vi "CAN GPS Werte.vi"() -> (2 "CAN data":T1[](array[typedef])=[{"timestamp"=timestamp(0 s since 1904-01-01), "payload"=[0, 2, 3, 4, 5, 6, 7, 8], "identifier"=2, "type"=0, "extended?"=FALSE, "echo?"=FALSE}, {"timestamp"=timestamp(0 s since 1904-01-01), "payload"=[0, 1, 2, 3, 4, 5, 6, 7], "identifier"=3, "type"=0, "extended?"=FALSE, "echo?"=FALSE}] {"payload" format="%x"; "timestamp" format="%<%.7X\n%x>T"; "type" items=["CAN Data"=0, "CAN Remote"=1, "CAN Bus Error"=2, "CAN 2.0 Data"=8, "CAN FD Data"=16, "CAN FD+BRS Data"=24, "J1939 Data"=192, "Delay"=224, "Log Trigger"=225, "Start Trigger"=226]; "identifier" format="%x"})   [LabVIEW 2020]
uses:
  <vilib>/xnet/xnet.llb/XNET Frame CAN.ctl
  <vilib>/xnet/xnet.llb/XNET Frame Type CAN.ctl
  FGV CAN Daten Aktionen.ctl
  Allgemein/Aktion FGV GPS.ctl
  CAN Interface.lvlib
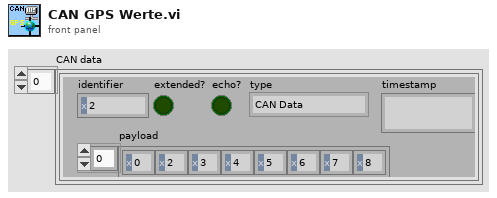
[diagram p1: front panel]
types:
  T1 = typedef "XNET Frame CAN.ctl" = cluster{"timestamp":timestamp, "payload":u8[], "identifier":u32, "type":T2, "extended?":bool, "echo?":bool}
  T2 = typedef "XNET Frame Type CAN.ctl" = u8
  T3 = typedef "Allgemein.lvlib/Aktion FGV GPS.ctl" = enum16{"lesen", "schreiben"}
  T4 = typedef "CAN Interface.lvlib/FGV CAN Daten Aktionen.ctl" = enum16{"lesen", "Daten", "Konfig", "laden", "speichern", "Status"}
  T5 = typedef "Allgemein.lvlib/GPS Daten cRio.ctl" = cluster{"GPS Zeit":string, "Breitengrad":string, "Längengrad":string, "Qualität":string, "Anzahl Satelliten":string, "Genauigkeit":string, "Höhe":string, "Höhe Geoid-Ellipsoid":string, "Geschwindigkeit":string, "Kurs wahr":string, "Kurs magnetisch":string, "Bewegungsrichtung":string, "Datum":string, "Breitengrad Roh":string, "Längengrad Roh":string}
  T6 = typedef "CAN Konfig.lvlib/Konfig Daten PC.ctl" = cluster{"Baude Rate":T7, "COM state":u8, "Frame-ID FTIR Start":u32, "Frame-ID FTIR End":u32, "Frame-ID Status Start":u32, "Frame-ID Status End":u32, "Zustand Information":u32, "Aktion":u32, "Frame-ID FTIR Arry":u32[], "Frame-ID Status Arry":u32[], "GPS Start":u32, "Interface":refnum<k21>}
  T7 = typedef "CAN Interface.lvlib/Baude Rate.ctl" = u32
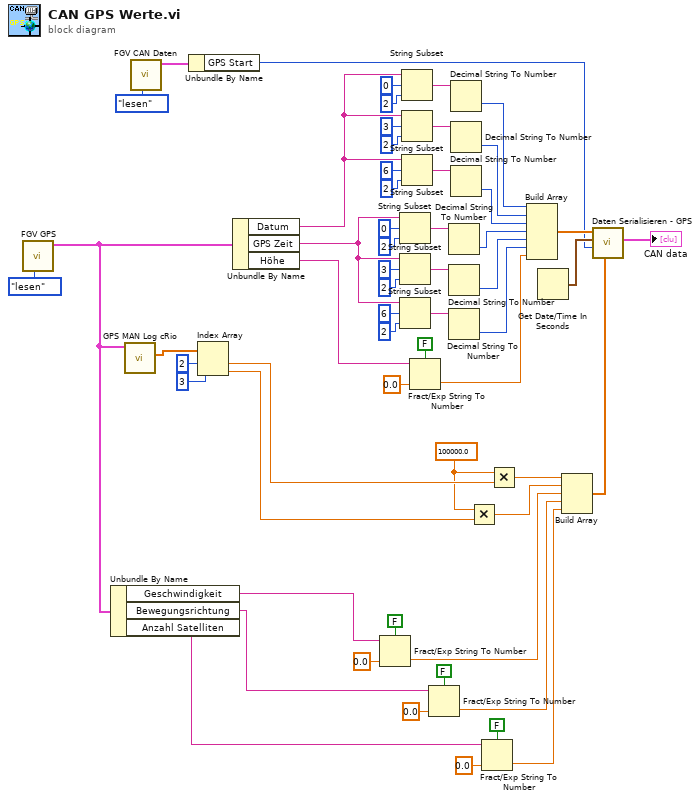
[diagram p0: block diagram]
diagram:
  w5 = sgl 100000.0 ("x")
  n1 = call "FGV GPS.vi"("Aktion"=Aktion_FGV_GPS."lesen") -> ("GPS Daten"=w16:T5)  [unwired: 10 in]
  n2 = Unbundle By Name(w16) -> ("Geschwindigkeit"=w25:string, "Bewegungsrichtung"=w26:string, "Anzahl Satelliten"=w18:string)
  n3 = call "GPS MAN Log cRio.vi"("Eingangs-Cluster"=w16) -> ("Array"=w15:sgl[])  [unwired: 8 in, 1 out]
  n4 = call "FGV CAN Daten.vi"("Aktionen"=FGV_CAN_Daten_Aktionen."lesen") -> ("Konfig Daten"=w59:T6)  [unwired: 8 in, 2 out]
  n5 = Unbundle By Name(w59) -> ("GPS Start"=w27:u32)
  n6 = Index Array(array=w15, index #1=2 ("Index"), index #2=3 ("Index")) -> (element #1=w20:sgl, element #2=w19:sgl)
  n7 = Unbundle By Name(w16) -> ("Datum"=w2:string, "GPS Zeit"=w1:string, "Höhe"=w33:string)
  n8 = Fract/Exp String To Number(use system decimal point (T)=FALSE ("Systemdezimalzeichen verwenden (T)"), string=w25, default (0 dbl)=sgl 0.0 ("Standard (0 DBL)")) -> (number=w4:sgl)  [unwired: 1 in, 1 out]
  n9 = String Subset(string=w1, offset (0)=0 ("Offset (0)"), length (rest)=2 ("Länge (Rest)")) -> (substring=w45:string)
  n10 = String Subset(string=w1, offset (0)=3 ("Offset (0)"), length (rest)=2 ("Länge (Rest)")) -> (substring=w46:string)
  n11 = String Subset(string=w1, offset (0)=6 ("Offset (0)"), length (rest)=2 ("Länge (Rest)")) -> (substring=w47:string)
  n12 = String Subset(string=w2, offset (0)=0 ("Offset (0)"), length (rest)=2 ("Länge (Rest)")) -> (substring=w51:string)
  n13 = String Subset(string=w2, offset (0)=3 ("Offset (0)"), length (rest)=2 ("Länge (Rest)")) -> (substring=w50:string)
  n14 = String Subset(string=w2, offset (0)=6 ("Offset (0)"), length (rest)=2 ("Länge (Rest)")) -> (substring=w49:string)
  n15 = Fract/Exp String To Number(use system decimal point (T)=FALSE ("Systemdezimalzeichen verwenden (T)"), string=w33, default (0 dbl)=sgl 0.0 ("Standard (0 DBL)")) -> (number=w30:sgl)  [unwired: 1 in, 1 out]
  n16 = Fract/Exp String To Number(use system decimal point (T)=FALSE ("Systemdezimalzeichen verwenden (T)"), string=w26, default (0 dbl)=sgl 0.0 ("Standard (0 DBL)")) -> (number=w3:sgl)  [unwired: 1 in, 1 out]
  n17 = Decimal String To Number(string=w45) -> (number=w38:i32)  [unwired: 2 in, 1 out]
  n18 = Decimal String To Number(string=w46) -> (number=w37:i32)  [unwired: 2 in, 1 out]
  n19 = Decimal String To Number(string=w47) -> (number=w36:i32)  [unwired: 2 in, 1 out]
  n20 = Decimal String To Number(string=w51) -> (number=w34:i32)  [unwired: 2 in, 1 out]
  n21 = Decimal String To Number(string=w50) -> (number=w48:i32)  [unwired: 2 in, 1 out]
  n22 = Decimal String To Number(string=w49) -> (number=w35:i32)  [unwired: 2 in, 1 out]
  n23 = Multiply(x=w5, y=w19) -> (x*y=w6:sgl)
  n24 = Fract/Exp String To Number(use system decimal point (T)=FALSE ("Systemdezimalzeichen verwenden (T)"), string=w18, default (0 dbl)=sgl 0.0 ("Standard (0 DBL)")) -> (number=w8:sgl)  [unwired: 1 in, 1 out]
  n25 = Multiply(x=w5, y=w20) -> (x*y=w7:sgl)
  n26 = Build Array(w34, w48, w35, w38, w37, w36, w30) -> (w29:sgl[])
  n27 = Get Date/Time In Seconds() -> (seconds since 1Jan1904=w28:timestamp)
  n28 = Build Array(w7, w6, w4, w3, w8) -> (w24:sgl[])
  n29 = call "Daten Serialisieren - GPS.vi"("GPS Position"=w24, "Frame-ID"=w27, "Aktuelle Zeit"=w28, "GPS Datum & Zeit"=w29) -> ("data"=→"CAN data":T1[])  [unwired: 7 in]
